vi "Launch Aircraft.vi"(8 "Error In":errorcluster) -> (0 "error out":errorcluster)   [LabVIEW 2014]
uses:
  Aircraft Information/Sub VI/Selected Aircraft/SubVI/Get Selected Aircraft.vi
  Commands/MAV_CMD Sub VI/MAV_CMD_MISSION_START.vi
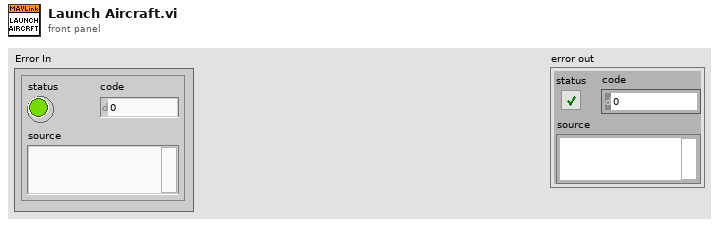
[diagram p1: front panel]
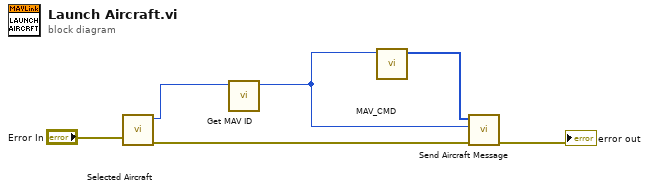
[diagram p0: block diagram]
diagram:
  n1 = call-poly "Selected Aircraft.vi"("Error In"="Error In") -> ("Error Out"=w4:errorcluster, "Selected Aircraft ID Out"=w5:u8)  [unwired: 9 in]
  n2 = call "Get MAV ID.vi"("Aircraft Index"=w5) -> ("Aircraft ID"=w3:u8)  [unwired: 9 in, 1 out]
  n3 = call-poly "MAV_CMD.vi"("Target System and Target Component"=w3) -> ("MAVLink Message"=w6:u8[])  [unwired: 10 in]
  n4 = call "Send Aircraft Message.vi"("error in (no error)"=w4, "Aircraft ID"=w3, "MAVLink Message"=w6) -> ("error out"=→"error out":errorcluster)  [unwired: 8 in]
